vi "Send-message.vi"(8 "error in (no error)":errorcluster, 9 "Receivers":string[](array[string]), 10 "Message":refnum<class "Message.lvclass">, 11 "Client in":T1) -> (0 "error out":errorcluster, 3 "Client out":T1)   [LabVIEW 2013, in "PowderDeposition.lvlib" / "PD-Client.lvclass"]
doc: "Send a message to the specified list of receivers.\nThe message is added to the back of the server message queue for processing.\nThe message needs to be created beforehand, either manually or through the 'Create-message' function and any specific contents need to be pre-configured. This function takes care of the sender and time information.\nThe receivers must be provided as an array. Each receiver entry can be composed in two ways: either '<module type>' to send to all active clients of the specified type, or '<module type><module ID>' to send to a specific client. Optionally the special client types 'All' or 'Server' can be used to send the message to all active clients (server excluded) or to the server, respectively."
uses:
  PD-Client.lvclass
  Object-reference.ctl
  SA-SLMAPI/Sources/Message.lvclass
  PD-Client.lvclass/PD-Client.ctl
  Main/PD-Main.lvclass
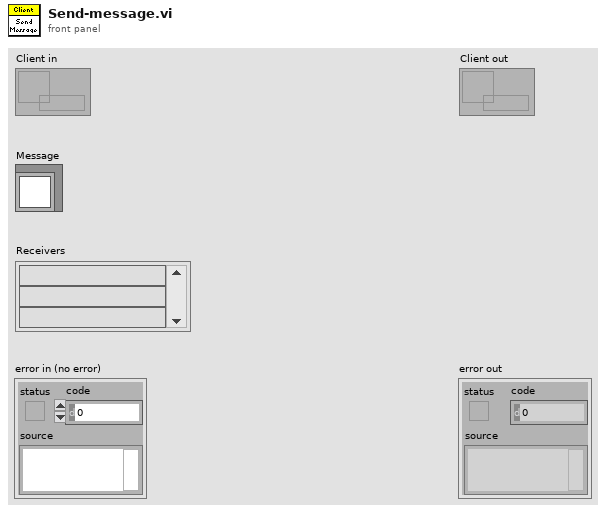
[diagram p1: front panel]
types:
  T1 = typedef "PowderDeposition.lvlib/PD-Client.lvclass/Object-reference.ctl" = refnum<data-value>
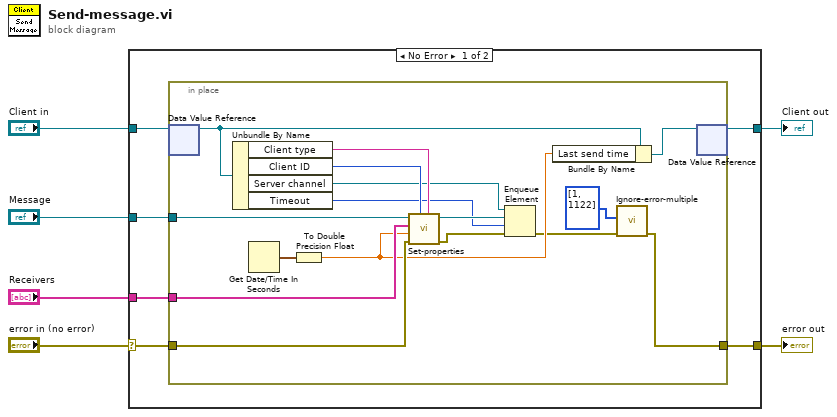
[diagram p0: block diagram]
diagram:
  n1 = case shown="No Error" "error in (no error)" {
    selector: "error in (no error)" -> [w8 w30]
    tunnel: [w7 w30] -> w5
    tunnel: [w9 w29] -> w3
    tunnel: "Client in" -> [w10 w29]
    tunnel: "Message" -> [w12 _]
    tunnel: "Receivers" -> [w11 _]
    frame No Error {
      n2 = in-place {
        in-place-border: w12 -> [w28]
        in-place-border: w11 -> [w27]
        in-place-border: w8 -> [w25]
        in-place-border: [w13] -> w7
        n3 = in-place-dvr #1(w10) -> (w19:refnum<class "PD-Client.lvclass">)  [unwired: 1 out]
        n4 = Unbundle By Name(w19) -> ("Client type"=w23:string, "Client ID"=w24:i32, "Server channel"=w20:refnum<queue>, "Timeout"=w21:i32)
        n5 = Get Date/Time In Seconds() -> (seconds since 1Jan1904=w26:timestamp)
        n6 = To Double Precision Float(number=w26) -> (double precision float=w17:dbl)
        n7 = call-dynamic "Set-properties.vi"("Sender type"=w23, "Sender ID"=w24, "error in (no error)"=w25, "Send time"=w17, "Receivers"=w27, "Message in"=w28) -> ("error out"=w14:errorcluster, "Message out"=w22:refnum<class "Message.lvclass">)  [unwired: 4 in]
        n8 = Enqueue Element(queue=w20, element=w22, timeout in ms (-1)=w21, error in (no error)=w14) -> (error out=w16:errorcluster)  [unwired: 2 out]
        n9 = Bundle By Name(cluster=w19, "Last send time"=w17) -> (w18:refnum<class "PD-Client.lvclass">)
        n10 = call "Ignore-error-multiple.vi"("error in (no error)"=w16, "Errors to ignore (1)"=i32[] [1, 1122]) -> ("error out"=w13:errorcluster)  [unwired: 9 in]
        n11 = in-place-dvr #1(w18) -> (w9:T1)  [unwired: 1 out]
      }
    }
    frame Error {
    }
  }
  "error out" <- w5
  "Client out" <- w3
